vi "PhotodiodeTest.vi"() -> ()   [LabVIEW 2020]
panel:
  in  "Time Step":i64
  in  "Number of Samples 2":i32=100
  out "Voltage from photodiode":dynamicdata(graph)
  out "Photo Resistor Value":dbl
  in  "stop":bool
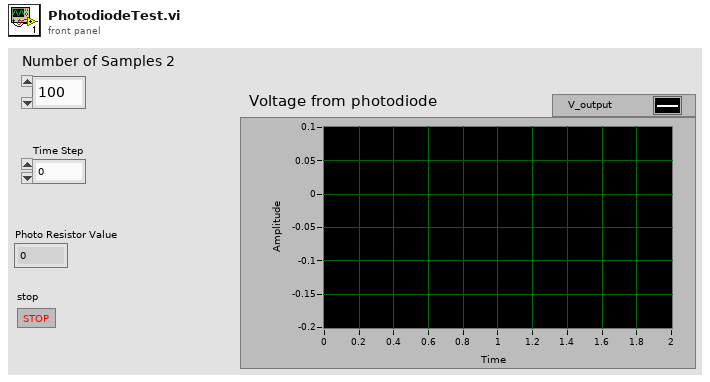
[diagram p1: front panel]
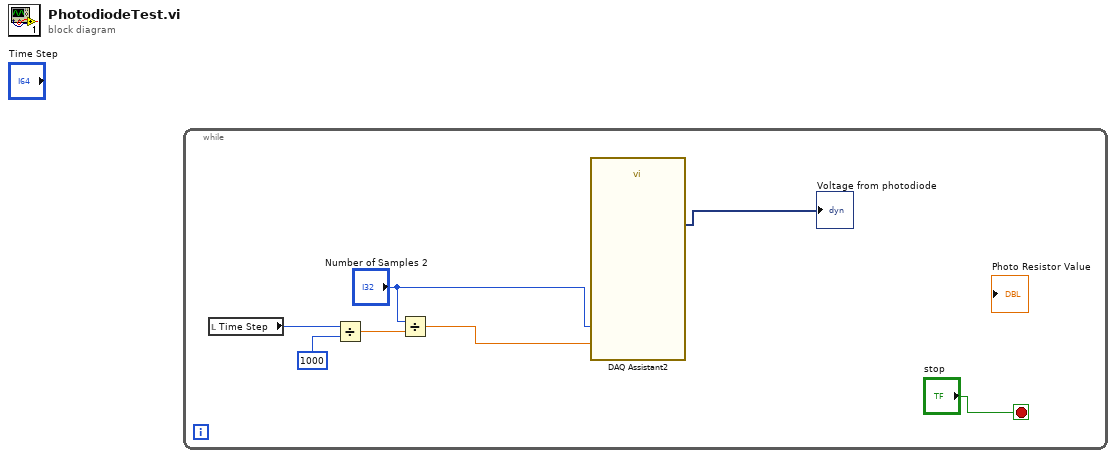
[diagram p0: block diagram]
diagram:
  n1 = while {
    stop <- "stop" stop-if-true
    n2 = local read "Time Step"() -> (w5:i64)
    n3 = Divide(x=w5, y=i64 1000) -> (x/y=w4:dbl)
    n4 = Divide(x="Number of Samples 2", y=w4) -> (x/y=w1:dbl)
    n5 = call "DAQ Assistant2"("rate"=w1, "number of samples"="Number of Samples 2") -> ("data"=→"Voltage from photodiode":dynamicdata)  [unwired: 3 in, 14 out]
  }
